vi "Report Core.vi"(8 "error in":errorcluster, 9 "Received":path, 10 "Approved":path, 11 "Report With Beyond Compare in":refnum<class "Report With Beyond Compare.lvclass">) -> (0 "error out":errorcluster, 2 "Worked?":bool, 3 "Report With Beyond Compare out":refnum<class "Report With Beyond Compare.lvclass">)   [LabVIEW 2020, in "Approval Tests.lvlib" / "Report With Beyond Compare.lvclass"]
uses:
  Report With Beyond Compare.lvclass
  Report With Beyond Compare.lvclass/Report With Beyond Compare.ctl
  Approval Tests.lvlib
  OS Strings.ctl
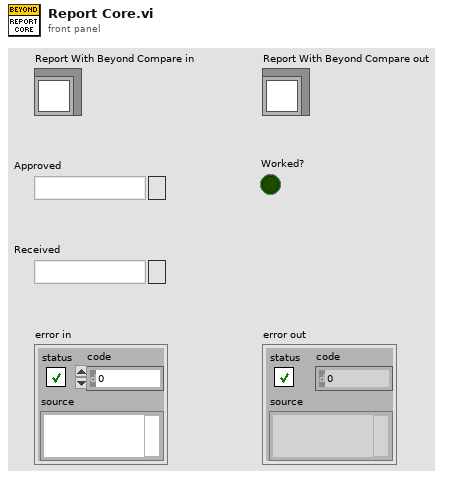
[diagram p1: front panel]
types:
  T1 = typedef "Approval Tests.lvlib/OS Strings.ctl" = cluster{"Windows":string, "Linux":string, "Mac":string}
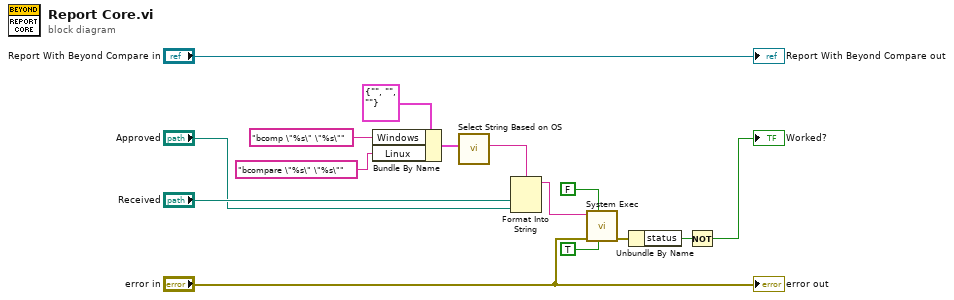
[diagram p0: block diagram]
diagram:
  n1 = Bundle By Name(cluster=T1 {"Windows"="", "Linux"="", "Mac"=""} ("Strings"), "Windows"="bcomp \"%s\" \"%s\"" ("format string"), "Linux"="bcompare \"%s\" \"%s\"" ("format string")) -> (w4:T1)
  n2 = call "Select String Based on OS.vi"("Strings"=w4) -> ("Selection"=w2:string)  [unwired: 10 in]
  n3 = Format Into String(format string=w2, "Received", "Approved") -> (resulting string=w12:string)  [unwired: 2 in, 1 out]
  n4 = call <vilib>:"System Exec.vi"("run minimized? (F)"=TRUE, "wait until completion? (T)"=FALSE, "error in (no error)"="error in", "command line"=w12) -> ("error out"=w15:errorcluster)  [unwired: 4 in, 3 out]
  n5 = Unbundle By Name(w15) -> ("status"=w8:bool)
  n6 = Not(x=w8) -> (.not. x?=→"Worked?":bool)
  "error out" <- "error in"
  "Report With Beyond Compare out" <- "Report With Beyond Compare in"
